vi "Dispose.vi"(8 "error in (no error)":errorcluster, 11 "Agent Fixture in":refnum<class "Agent Fixture.lvclass">) -> (0 "error out":errorcluster)   [LabVIEW 2013, in "libssh2_integration_tests.lvlib" / "Agent Fixture.lvclass"]
uses:
  Agent Fixture.lvclass
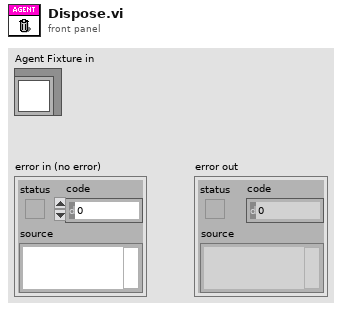
[diagram p1: front panel]
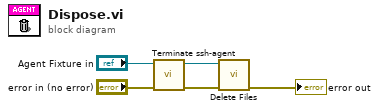
[diagram p0: block diagram]
diagram:
  n1 = call "Terminate ssh-agent.vi"("error in (no error)"="error in (no error)", "Agent Fixture in"="Agent Fixture in") -> ("error out"=w4:errorcluster, "Agent Fixture out"=w1:refnum<class "Agent Fixture.lvclass">)  [unwired: 6 in, 2 out]
  n2 = call "Delete Files.vi"("error in (no error)"=w4, "Agent Fixture in"=w1) -> ("error out"=→"error out":errorcluster)  [unwired: 8 in, 1 out]
